vi "Get Possibilities.vi"(1 "Damaged Springs":i32[](array[numeric]), 2 "Spring Record":string) -> (0 "Possible Spring Records":string[](array[string]))   [LabVIEW 2020, in "AoC 2023.lvlib"]
uses:
  AoC 2023.lvlib
  <vilib>/regexp/Match Regular Expression.xnode
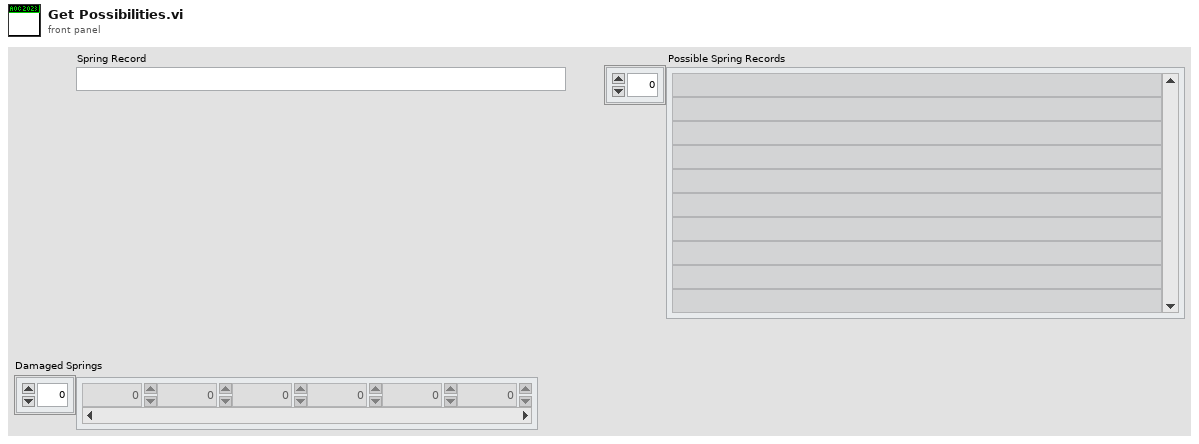
[diagram p1: front panel]
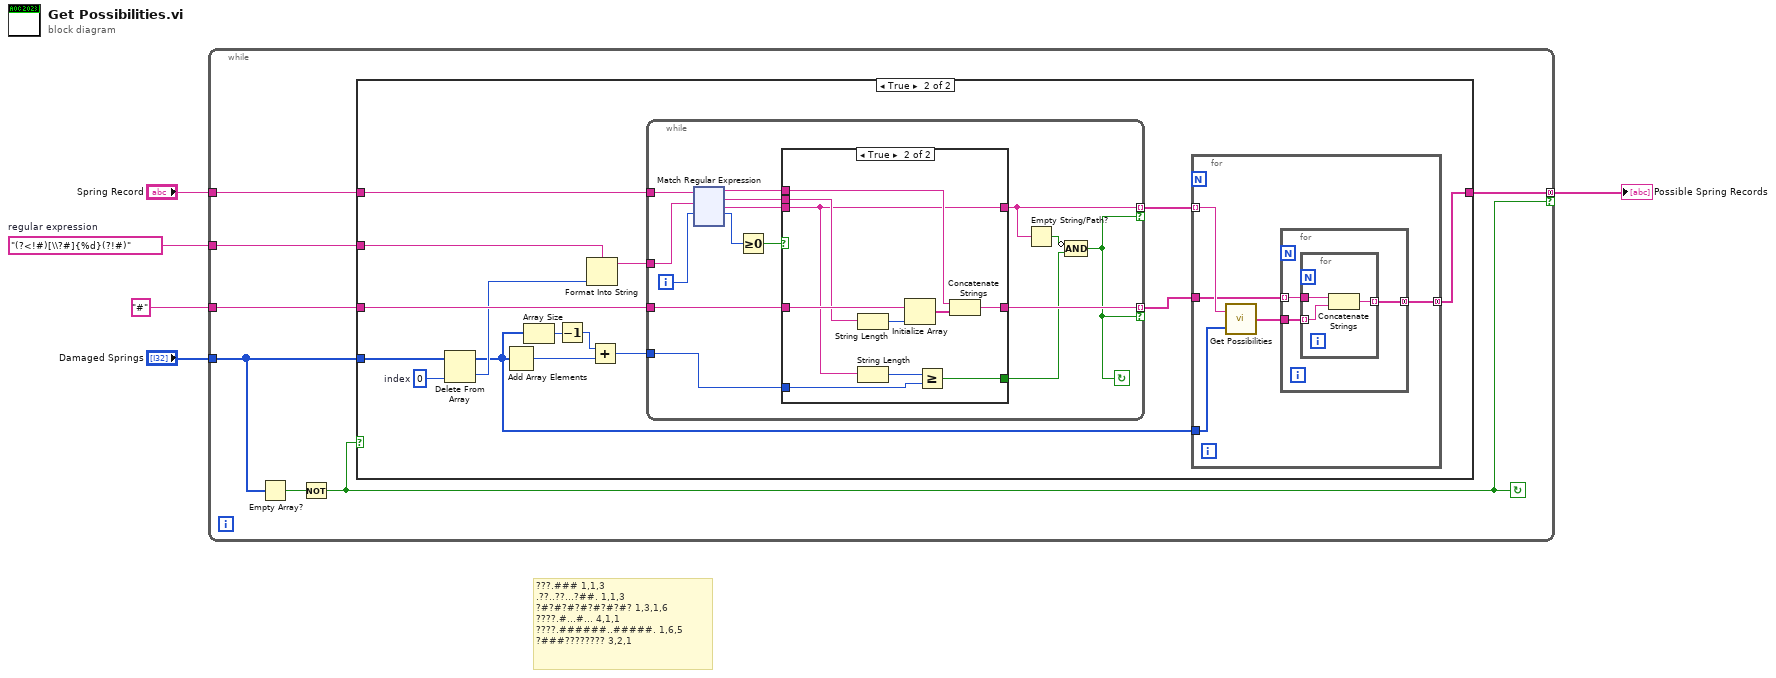
[diagram p0: block diagram]
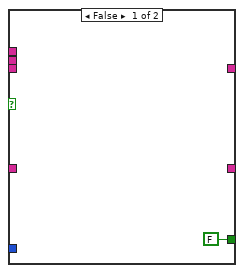
[diagram p3: hidden frame]
diagram:
  w2 = "(?<!#)[\\?#]{%d}(?!#)"  # regular expression
  # "???.### 1,1,3\n.??..??...?##. 1,1,3\n?#?#?#?#?#?#?#? 1,3,1,6\n????.#...#... 4,1,1\n????.######..#####. 1,6,5\n?###???????? 3,2,1"
  n1 = while {
    tunnel: w2 -> [w12]
    tunnel: "#" -> [w11]
    tunnel: [w8] -> w3 mode=concatenating if=w6
    tunnel: "Damaged Springs" -> [w9]
    tunnel: "Spring Record" -> [w10]
    stop <- w6 continue-if-true
    n2 = Empty Array?(array=w9) -> (empty?=w7:bool)
    n3 = Not(x=w7) -> (.not. x?=w6:bool)
    n4 = case shown="True" w6 {
      tunnel: w12 -> [_ w27]
      tunnel: w11 -> [_ w26]
      tunnel: w10 -> [_ w25]
      tunnel: w9 -> [_ w16]
      tunnel: [_ w15] -> w8
      frame False {
      }
      frame True {
        w18 = 0  # index
        n5 = Delete From Array(array=w16, index=w18) -> (deleted portion=w23:i32, array with subset deleted=w14:i32[])  [unwired: 1 in]
        n6 = Add Array Elements(numeric array=w14) -> (sum=w20:i32)
        n7 = Array Size(array=w14) -> (size(s)=w22:i32)
        n8 = Decrement(x=w22) -> (x-1=w21:i32)
        n9 = Format Into String(format string=w27, w23) -> (resulting string=w24:string)  [unwired: 2 in, 1 out]
        n10 = Add(x=w21, y=w20) -> (x+y=w19:i32)
        n11 = while {
          tunnel: w25 -> [w50]
          tunnel: w26 -> [w53]
          tunnel: w24 -> [w49]
          tunnel: [w52] -> w17 mode=indexing if=w39
          tunnel: w19 -> [w51]
          tunnel: [w42] -> w13 mode=indexing if=w39
          i -> [w48]
          stop <- w39 continue-if-true
          n12 = xnode "Match Regular Expression"("input string"=w50, "regular expression"=w49, "offset (0)"=w48) -> ("before match"=w47:string, "whole match"=w46:string, "after match"=w45:string, "offset past match"=w44:i32)  [unwired: 3 in, 1 out]
          n13 = Greater Or Equal To 0?(x=w44) -> (x >= 0?=w43:bool)
          n14 = case shown="True" w43 {
            tunnel: w53 -> [_ w63]
            tunnel: [_ w61] -> w52
            tunnel: w51 -> [_ w59]
            tunnel: w47 -> [_ w58]
            tunnel: w46 -> [_ w57]
            tunnel: w45 -> [_ w55]
            tunnel: [FALSE w56] -> w40
            tunnel: [_ w55] -> w42
            frame False {
            }
            frame True {
              n15 = String Length(string=w57) -> (length=w64:i32)
              n16 = String Length(string=w55) -> (length=w60:i32)
              n17 = Initialize Array(w63, w64) -> (w62:string[])
              n18 = Greater Or Equal?(x=w60, y=w59) -> (x >= y?=w56:bool)
              n19 = Concatenate Strings(w58, w62) -> (w61:string)
            }
          }
          n20 = Empty String/Path?(string/path=w42) -> (empty?=w41:bool)
          n21 = Compound Arithmetic op=AND(invert w41, w40) -> (w39:bool)
        }
        n22 = for {
          tunnel: w17 -> [w30]
          tunnel: w14 -> [w32]
          tunnel: [w28] -> w15 mode=concatenating
          tunnel: w13 -> [w31] mode=indexing
          n23 = call "Get Possibilities.vi"("Damaged Springs"=w32, "Spring Record"=w31) -> ("Possible Spring Records"=w29:string[])
          n24 = for {
            tunnel: w30 -> [w34] mode=indexing
            tunnel: w29 -> [w35]
            tunnel: [w33] -> w28 mode=concatenating
            n25 = for {
              tunnel: w35 -> [w37] mode=indexing
              tunnel: w34 -> [w38]
              tunnel: [w36] -> w33 mode=indexing
              n26 = Concatenate Strings(w38, w37) -> (w36:string)
            }
          }
        }
      }
    }
  }
  "Possible Spring Records" <- w3
